vi "Prepare Bus Monitor Interface.vi"(9 "Datum Name":string, 11 "IBusMonitor":refnum<class "IBusMonitor.lvclass">) -> (2 "Valid Transport":refnum<class "ITransport.lvclass">, 3 "SubscriptionPolicy":refnum<class "ISubscriptionPolicy.lvclass">)   [LabVIEW 2017, in "MonitoredMediator.lvlib" / "IBusMonitor.lvclass"]
doc: "<License>\nCopyright © 2020 Tymphany, LLC | All rights reserved\nwww.Tymphany.com\nHuijun <Huijun.Guo@Tymphany.com>\n</License>"
uses:
  <userlib>/composed/mva-core/Source/MonitoredMediator/IBusMonitor/IBusMonitor.lvclass
  <userlib>/composed/transport/Source/ITransport/ITransport.lvclass
  <userlib>/composed/mva-core/Source/IMediator/ISubscriptionPolicy/ISubscriptionPolicy.lvclass
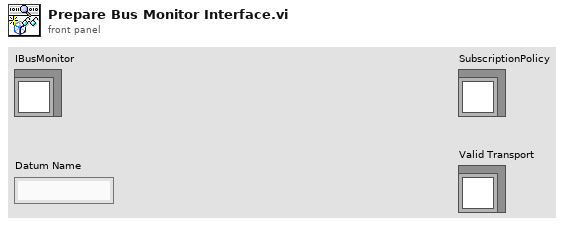
[diagram p1: front panel]
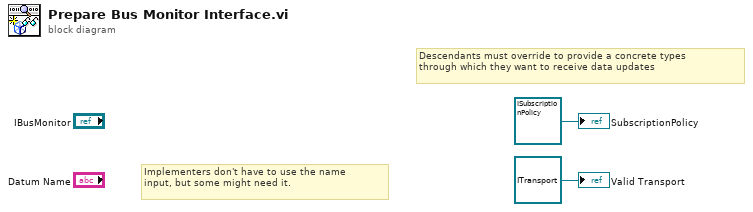
[diagram p0: block diagram]
diagram:
  # "Implementers don't have to use the name\ninput, but some might need it."
  # "Descendants must override to provide a concrete types\nthrough which they want to receive data updates"
  "Valid Transport" <- refnum<class "ITransport.lvclass"> refnum ("Notification Msg Type")
  "SubscriptionPolicy" <- refnum<class "ISubscriptionPolicy.lvclass"> refnum ("Bus Monitor SubscriptionPolicy")
